vi "CNT Init Counter.vi"(7 "pInitConfig":T1, 9 "Channel":u8, 10 "DevIndex":i32, 11 "DevType":i32) -> (3 "function return":i32, 5 "pInitConfig out":T1)   [LabVIEW 2010, in "ControlCNT.lvlib"]
doc: "int WINAPI CNT_InitCounter(int DevType, int DevIndex, unsigned char Channel, PCNT_INIT_CONFIG pInitConfig);"
uses:
  ControlCNT.lvlib
  ControlCNT/Ginkgo_Driver.dll
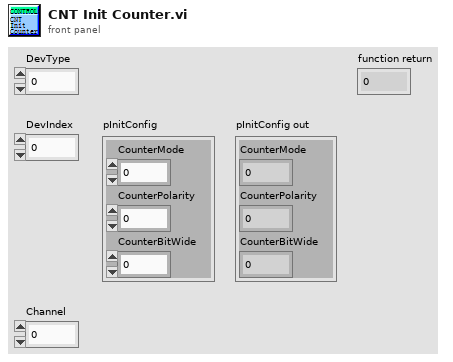
[diagram p1: front panel]
types:
  T1 = cluster{"CounterMode":u8, "CounterPolarity":u8, "CounterBitWide":u8}
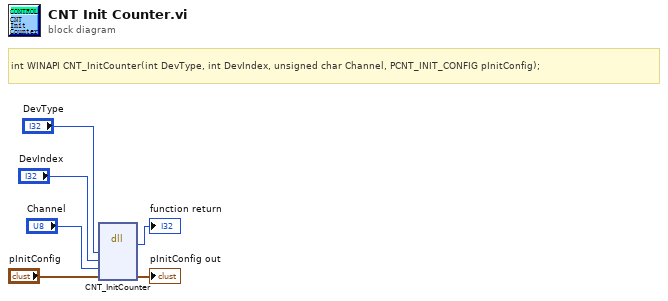
[diagram p0: block diagram]
diagram:
  # "int WINAPI CNT_InitCounter(int DevType, int DevIndex, unsigned char Channel, PCNT_INIT_CONFIG pInitConfig);"
  n1 = dll-call lib="E:/Project/vt_ginkgo/truck/Ginkgo Driver/vs2010/Ginkgo_USB-I2C&SPI&CAN_API_v2.0.3.3/lib/labview_32bit/ControlCNT/Ginkgo_Driver.*" fn="CNT_InitCounter"("DevType"="DevType", "DevIndex"="DevIndex", "Channel"="Channel", "pInitConfig"="pInitConfig") -> (→"function return":i32, "pInitConfig"=→"pInitConfig out":T1)  [unwired: 6 in, 2 out]
